vi "b_n__v1.vi"(0 "光線ベクトル[n-1]":ext[][](array[numeric]), 6 "D":ext, 8 "R":ext, 10 "n":ext) -> (14 "b[n]":ext)   [LabVIEW 2020]
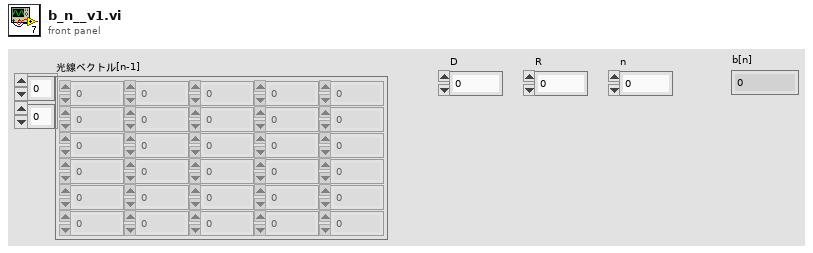
[diagram p1: front panel]
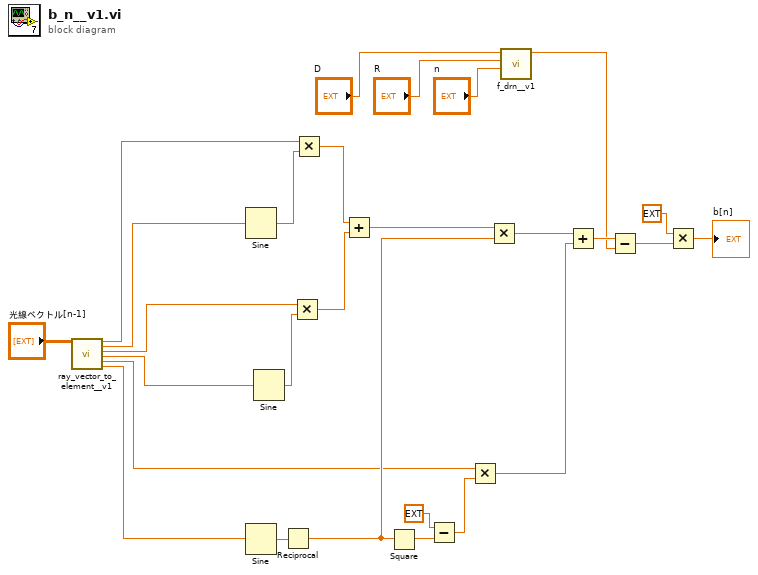
[diagram p0: block diagram]
diagram:
  n1 = call "ray_vector_to_element__v1.vi"("光線ベクトル"="光線ベクトル[n-1]") -> ("x"=w6:ext, "α"=w5:ext, "y"=w4:ext, "β"=w3:ext, "z"=w2:ext, "γ"=w1:ext)  [unwired: 13 in]
  n2 = Sine(x=w5) -> (sin(x)=w26:ext)
  n3 = Sine(x=w1) -> (sin(x)=w22:ext)
  n4 = Sine(x=w3) -> (sin(x)=w27:ext)
  n5 = Reciprocal(x=w22) -> (1/x=w12:ext)
  n6 = Multiply(x=w4, y=w27) -> (x*y=w24:ext)
  n7 = Multiply(x=w6, y=w26) -> (x*y=w25:ext)
  n8 = Add(x=w25, y=w24) -> (x+y=w11:ext)
  n9 = Square(x=w12) -> (x^2=w21:ext)
  n10 = Subtract(x=ext 1.0, y=w21) -> (x-y=w13:ext)
  n11 = Multiply(x=w2, y=w13) -> (x*y=w15:ext)
  n12 = Multiply(x=w11, y=w12) -> (x*y=w14:ext)
  n13 = call "f_drn__v1.vi"("n"="n", "R"="R", "D"="D") -> ("出力結果"=w9:ext)  [unwired: 8 in]
  n14 = Add(x=w14, y=w15) -> (x+y=w10:ext)
  n15 = Subtract(x=w10, y=w9) -> (x-y=w8:ext)
  n16 = Multiply(x=ext 2.0, y=w8) -> (x*y=→"b[n]":ext)
